vi "BuildDropNotice.vi"(8 "error in (no error)":errorcluster, 11 "droppeedCount":i32) -> (0 "error out":errorcluster, 3 "Statement":T1={"timestamp"=timestamp(0 s since 1904-01-01), "level"=enum."INFO", "sourceTag"="", "originVI"="", "message"=""})   [LabVIEW 2026, in "Lumberjack.lvlib"]
doc: "Builds the synthetic drop-notice Statement that an appender emits to make dropped-statement gaps visible (SRS-LMBR-059). Given the number of statements dropped since the last notice, it returns a Statement with message = \"dropped statement count = <N>\" (key=value form, so no singular/plural cases), level = ERROR, sourceTag = \"lumberjack.dropped\", and the timestamp stamped at build time.\nlevel = ERROR is deliberate: ERROR is protected, so a level-aware appender never sheds the notice itself. (The emission path in Actor Core also routes the notice straight to the sink, bypassing ApplyDropPolicy, so drop-oldest/drop-newest can't discard it either.) The \"lumberjack.*\" sourceTag namespace is reserved for Lumberjack's own system messages, letting consumers distinguish a system notice from a user log.\nSupport helper (src/Support/Backpressure), community scope; a pure field-builder (no state, no sink I/O), directly unit-testable (LMBR-T-051). Called by Appender.Actor Core when its dropped counter is non-zero at the emission point."
uses:
  Lumberjack.lvlib
  TypeDefs/Severity.ctl
  TypeDefs/Statement.ctl
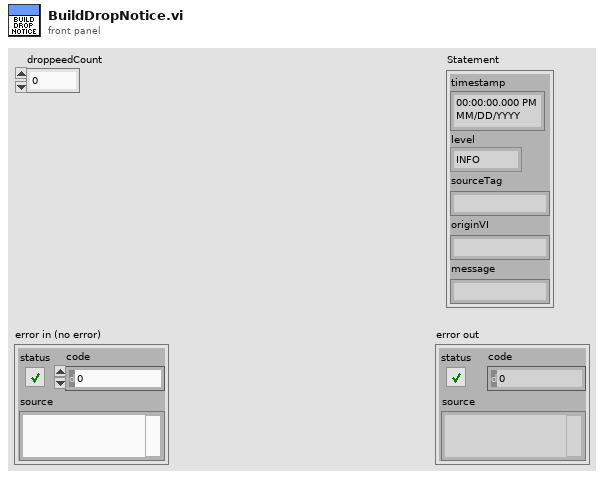
[diagram p1: front panel]
types:
  T1 = typedef "Lumberjack.lvlib/Statement.ctl" = cluster{"timestamp":timestamp, "level":T2, "sourceTag":string, "originVI":string, "message":string}
  T2 = typedef "Lumberjack.lvlib/Severity.ctl" = enum16{"OFF", "FATAL", "ERROR", "WARN", "INFO", "DEBUG", "TRACE", "ALL"}
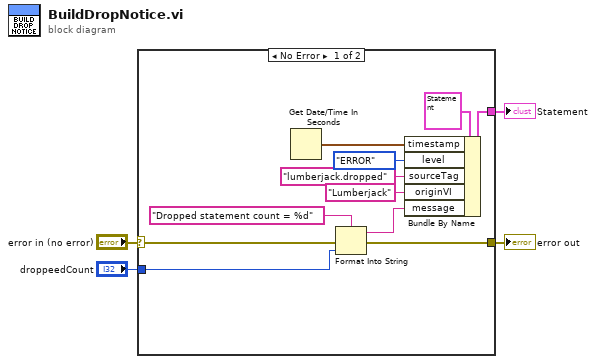
[diagram p0: block diagram]
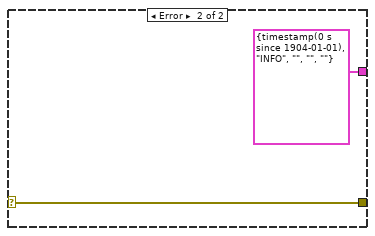
[diagram p2: hidden frame]
diagram:
  n1 = case shown="No Error" "error in (no error)" {
    selector: "error in (no error)" -> [w15 w17]
    tunnel: [w14 w17] -> w4
    tunnel: "droppeedCount" -> [w13 _]
    tunnel: [w11 T1 {"timestamp"=timestamp(0 s since 1904-01-01), "level"=enum."INFO", "sourceTag"="", "originVI"="", "message"=""} ("Statement")] -> w1
    frame No Error {
      n2 = Get Date/Time In Seconds() -> (seconds since 1Jan1904=w10:timestamp)
      n3 = Format Into String(format string="Dropped statement count = %d", error in=w15, w13) -> (resulting string=w6:string, error out=w14:errorcluster)  [unwired: 1 in]
      n4 = Bundle By Name(cluster=T1 {"timestamp"=timestamp(0 s since 1904-01-01), "level"=enum."INFO", "sourceTag"="", "originVI"="", "message"=""} ("Statement"), "timestamp"=w10, "level"=Severity."ERROR", "sourceTag"="lumberjack.dropped", "originVI"="Lumberjack", "message"=w6) -> (w11:T1)
    }
    frame Error {
    }
  }
  "error out" <- w4
  "Statement" <- w1
